vi "Vision Server Open.vi"(8 "error in (no error)":errorcluster, 10 "ADB Path (Optional)":path, 11 "port (8254)":u16=8254) -> (0 "error out":errorcluster, 3 "VisionServerRef out":T1)   [LabVIEW 2016, in "Vision Server.lvclass"]
uses:
  Vision Server.lvclass
  typedef/Vision Server Ref.ctl
  typedef/Message Type.ctl
  Vision Server.lvclass/Vision Server.ctl
  AdbBridge/Adb Bridge.lvclass
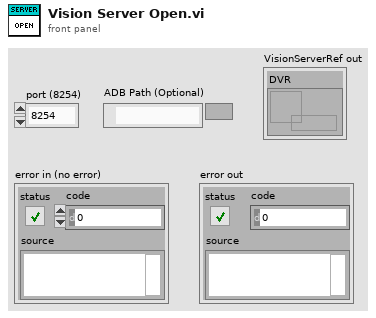
[diagram p1: front panel]
types:
  T1 = typedef "Vision Server.lvclass/Vision Server Ref.ctl" = cluster{"DVR":refnum<data-value>}
  T2 = typedef "Vision Server.lvclass/Message Type.ctl" = cluster{"type":string, "message":string}
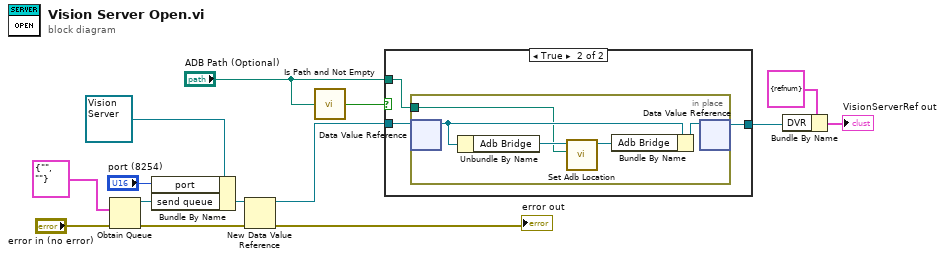
[diagram p0: block diagram]
diagram:
  n1 = Obtain Queue(element data type=T2 {"type"="", "message"=""} ("Cluster"), error in (no error)="error in (no error)") -> (queue out=w11:refnum<queue>, error out=w14:errorcluster)  [unwired: 3 in, 1 out]
  n2 = Bundle By Name(cluster=refnum<class "Vision Server.lvclass"> refnum ("Vision Server.lvclass"), "port"="port (8254)", "send queue"=w11) -> (w13:refnum<class "Vision Server.lvclass">)
  n3 = New Data Value Reference(data value=w13, error in=w14) -> (data value reference=w2:refnum<data-value>, error out=→"error out":errorcluster)
  n4 = call <vilib>:"Is Path and Not Empty.vi"("path"="ADB Path (Optional)") -> ("Is Path and Not Empty?"=w4:bool)  [unwired: 4 in]
  n5 = case shown="True" w4 {
    tunnel: w2 -> [w15 w18]
    tunnel: [w15 w17] -> w1
    tunnel: "ADB Path (Optional)" -> [_ w16]
    frame False {
    }
    frame True {
      n6 = in-place {
        in-place-border: w16 -> [w19]
        n7 = in-place-dvr #1(w18) -> (w22:refnum<class "Vision Server.lvclass">)  [unwired: 1 out]
        n8 = Unbundle By Name(w22) -> ("Adb Bridge"=w21:refnum<class "Adb Bridge.lvclass">)
        n9 = call "Set Adb Location.vi"("adb path"=w19, "AdbBridge in"=w21) -> ("AdbBridge out"=w20:refnum<class "Adb Bridge.lvclass">)  [unwired: 8 in, 1 out]
        n10 = Bundle By Name(cluster=w22, "Adb Bridge"=w20) -> (w23:refnum<class "Vision Server.lvclass">)
        n11 = in-place-dvr #1(w23) -> (w17:refnum<data-value>)  [unwired: 1 out]
      }
    }
  }
  n12 = Bundle By Name(cluster=T1 {"DVR"=refnum} ("VisionServerRef out"), "DVR"=w1) -> (→"VisionServerRef out":T1)
